vi "Enable Current Sharing.vi"(8 "error in (no error)":errorcluster, 11 "69X_79X in":refnum<class "79XRP.lvclass">) -> (0 "error out":errorcluster, 3 "69X_79X out":refnum<class "79XRP.lvclass">)   [LabVIEW 2019]
uses:
  79XRP.lvclass
  C:/Users/Public/Documents/Development/builds/Instruments/PowerSupply.lvlibp/Library/PowerSupply.lvclass
  C:/Users/Public/Documents/Development/builds/Instruments/Instruments.lvlibp/Library/Instruments.lvclass
  C:/Users/Public/Documents/Development/builds/Tools/Config.lvlibp/Config.lvclass
  C:/Users/Public/Documents/Development/builds/Engine/Engine.lvlibp/Project/Engine.lvclass
  C:/Users/Public/Documents/Development/builds/Engine/Panel Manager.lvlibp/Panel Actor/Panel Actor.lvclass
  C:/Users/Public/Documents/Development/builds/Engine/Monitored Actor.lvlibp/Monitored Actor/Monitored Actor/Monitored Actor.lvclass
  C:/Users/Public/Documents/Development/builds/Engine/Actor Framework.lvlibp/1abvi3w/vi.lib/ActorFramework/Actor/Actor.lvclass
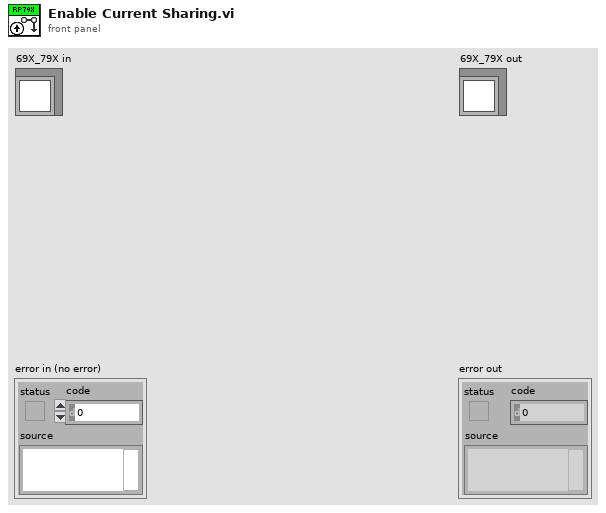
[diagram p1: front panel]
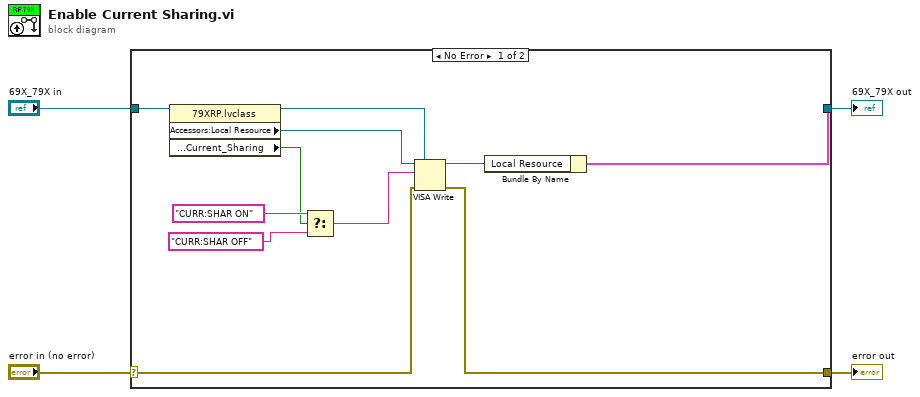
[diagram p0: block diagram]
diagram:
  n1 = case shown="No Error" "error in (no error)" {
    selector: "error in (no error)" -> [w13 w17]
    tunnel: [w12 w17] -> w3
    tunnel: [w15 w16] -> w1
    tunnel: "69X_79X in" -> [w11 w16]
    frame No Error {
      n2 = property class="79XRP.lvclass"(reference=w11) -> (reference out=w10:refnum<class "79XRP.lvclass">, "Accessors:Local Resource"=w9:refnum<visa-resource-name>, "Accessors:Setting:Current_Sharing"=w6:bool)  [unwired: 1 in, 1 out]
      n3 = Select(t="CURR:SHAR ON" ("write buffer"), s=w6, f="CURR:SHAR OFF" ("write buffer")) -> (s? t:f=w7:string)
      n4 = VISA Write(VISA resource name=w9, write buffer=w7, error in (no error)=w13) -> (VISA resource name out=w14:refnum<visa-resource-name>, error out=w12:errorcluster)  [unwired: 1 out]
      n5 = Bundle By Name(cluster=w10, "Local Resource"=w14) -> (w15:cluster{})
    }
    frame Error {
    }
  }
  "error out" <- w3
  "69X_79X out" <- w1
